vi "Configure View Model.vi"(8 "error in (no error)":errorcluster, 10 "List Box View Model":refnum<class "List Box View Model.lvclass">, 11 "List Box View In":refnum<class "Processes List Box View.lvclass">) -> (0 "error out":errorcluster, 3 "List Box View Out":refnum<class "Processes List Box View.lvclass">)   [LabVIEW 2020, in "Processes List Box View.lvclass"]
uses:
  Processes List Box View.lvclass
  List Box View Model_/List Box View Model.lvclass
  Processes List Box View.lvclass/Processes List Box View.ctl
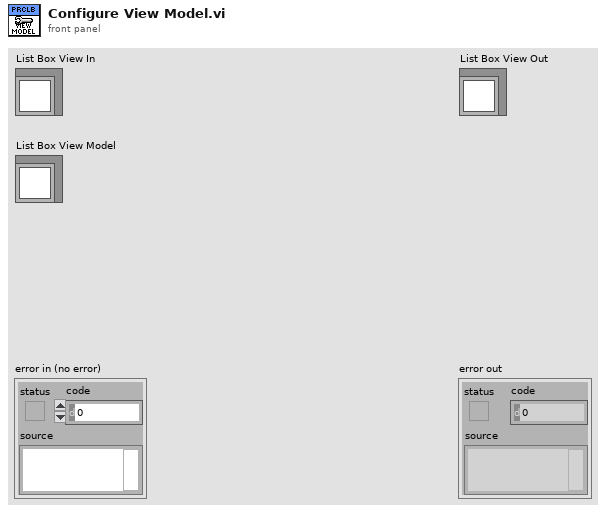
[diagram p1: front panel]
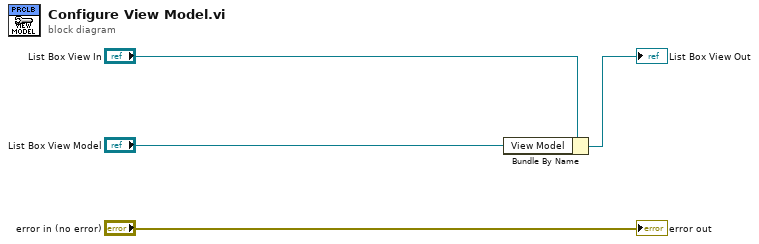
[diagram p0: block diagram]
diagram:
  n1 = Bundle By Name(cluster="List Box View In", "View Model"="List Box View Model") -> (→"List Box View Out":refnum<class "Processes List Box View.lvclass">)
  "error out" <- "error in (no error)"
